vi "Send to Alice.vi"(8 "error in (no error)":errorcluster, 11 "Bob in":refnum<class "Bob.lvclass">) -> (0 "error out":errorcluster, 3 "Bob out":refnum<class "Bob.lvclass">)   [LabVIEW 2014, in "Bob.lvlib" / "Bob.lvclass"]
uses:
  Bob.lvclass
  Bob.lvclass/Bob.ctl
  <vilib>/ActorFramework/Message Enqueuer/Message Enqueuer.lvclass/Message Enqueuer.ctl
  <vilib>/ActorFramework/Message Enqueuer/Enqueue.vi
  <vilib>/ActorFramework/Message Priority Queue/Priority Enqueue.vi
  Alice/Alice Messages/Alice Action Msg/Alice Action Msg.lvclass
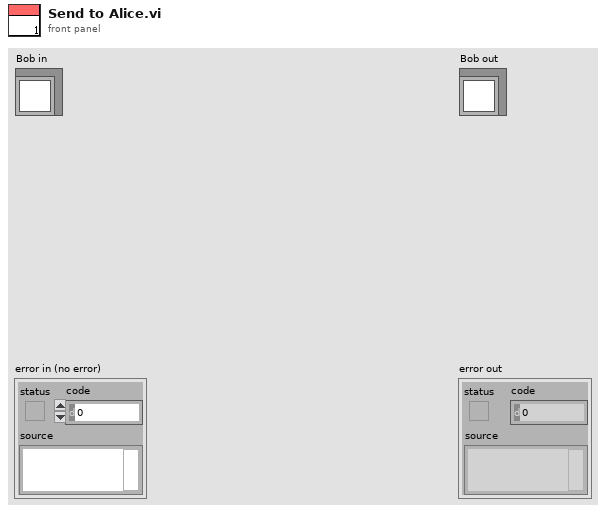
[diagram p1: front panel]
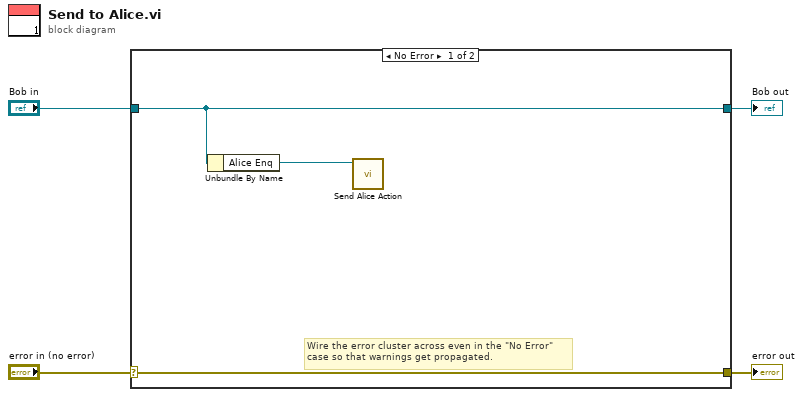
[diagram p0: block diagram]
diagram:
  n1 = case shown="No Error" "error in (no error)" {
    selector: "error in (no error)" -> [w7 w9]
    tunnel: [w7 w9] -> w3
    tunnel: [w6 w8] -> w1
    tunnel: "Bob in" -> [w6 w8]
    frame No Error {
      # "Wire the error cluster across even in the \"No Error\"\ncase so that warnings get propagated."
      n2 = Unbundle By Name(w6) -> ("Alice Enq"=w5:refnum<class "Message Enqueuer.lvclass">)
      n3 = call "Send Alice Action.vi"("Message Enqueuer"=w5) -> ()  [unwired: 9 in, 2 out]
    }
    frame Error {
    }
  }
  "error out" <- w3
  "Bob out" <- w1
